vi "PicoScope5000aGetTimebase2.vi"(4 "Number of Samples":u32, 6 "Memory Segment":u32, 7 "Acquisition Settings":T2={"preTriggerSamples"=0, "postTriggerSamples"=1000, "timebase"=2, "Down-Sample Mode"=0, "Down Sample Ratio"=1} {"Down Sample Ratio" min=1 step=1; "Down-Sample Mode" items=["None"=0, "Aggregate"=1, "Decimate"=2, "Average"=4]}, 10 "handle in":i16, 11 "error in (no error)":errorcluster) -> (2 "handle out":i16, 3 "error out":errorcluster, 5 "Properties Panel":T1 {"Max Total Capture Time Available (sec)" format="%.3p"; "Sample Frequency" format="%.3p"; "Sample Rate" format="%.3p"; "Max Samples Available" format="%.3p"; "Total Capture Time (sec)" format="%.3p"})   [LabVIEW 2020]
uses:
  ps5000a.dll
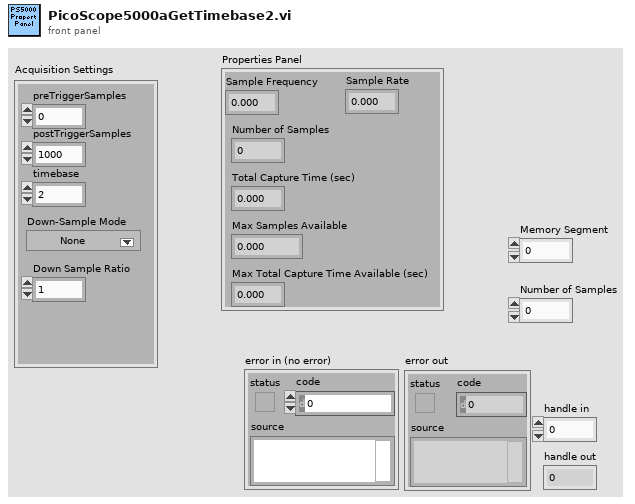
[diagram p1: front panel]
types:
  T1 = cluster{"Sample Frequency":sgl, "Sample Rate":sgl, "Max Samples Available":i32, "Number of Samples":u32, "Total Capture Time (sec) ":sgl, "Max Total Capture Time Available (sec)":sgl}
  T2 = cluster{"preTriggerSamples":i32, "postTriggerSamples":i32, "timebase":u32, "Down-Sample Mode":u32, "Down Sample Ratio":u32}
  T3 = cluster{sgl, sgl, "maxSamples":i32, "Number of Samples":u32, sgl, sgl}
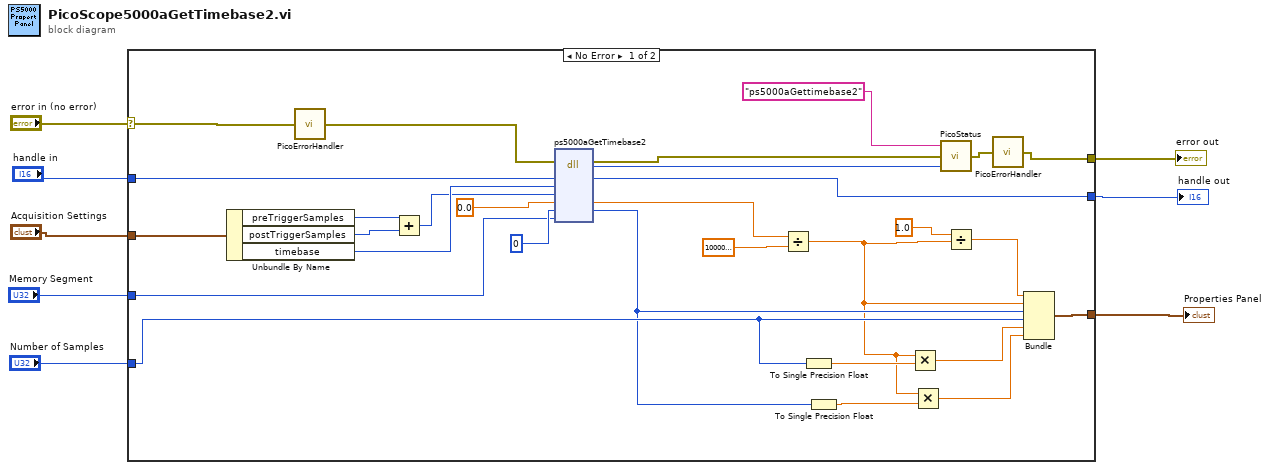
[diagram p0: block diagram]
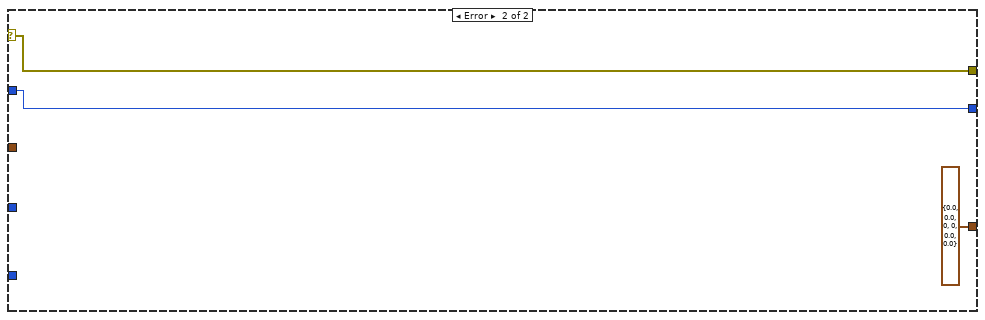
[diagram p2: hidden frame]
diagram:
  n1 = case shown="No Error" "error in (no error)" {
    selector: "error in (no error)" -> [w26 w40]
    tunnel: [w9 w40] -> w8
    tunnel: [w25 w39] -> w7
    tunnel: "Memory Segment" -> [w24 _]
    tunnel: "Number of Samples" -> [w18 _]
    tunnel: "handle in" -> [w23 w39]
    tunnel: "Acquisition Settings" -> [w22 _]
    tunnel: [w14 T3 {0.0, 0.0, "maxSamples"=0, "Number of Samples"=0, 0.0, 0.0}] -> w1
    frame No Error {
      n2 = Unbundle By Name(w22) -> ("preTriggerSamples"=w31:i32, "postTriggerSamples"=w32:i32, "timebase"=w33:u32)
      n3 = call "PicoErrorHandler.vi"("error in"=w26) -> ("error out"=w35:errorcluster)
      n4 = Add(x=w31, y=w32) -> (x+y=w20:i32)
      n5 = dll-call lib="ps5000a.dll" fn="ps5000aGetTimebase2"(error in=w35, "handle"=w23, "timebase"=w33, "noSamples"=w20, "timeIntervalNanoseconds"=sgl 0.0, "maxSamples"=0, "segmentIndex"=w24) -> (error out=w34:errorcluster, "PICO_STATUS"=w27:u32, "handle"=w25:i16, "timeIntervalNanoseconds"=w36:sgl, "maxSamples"=w16:i32)  [unwired: 5 in, 1 out]
      n6 = Divide(x=w36, y=sgl 1000000000.0) -> (x/y=w13:sgl)
      n7 = To Single Precision Float(number=w18) -> (single precision float=w21:sgl)
      n8 = To Single Precision Float(number=w16) -> (single precision float=w17:sgl)
      n9 = Multiply(x=w13, y=w21) -> (x*y=w19:sgl)
      n10 = Multiply(x=w13, y=w17) -> (x*y=w15:sgl)
      n11 = call "PicoStatus.vi"("PICO STATUS"=w27, "error in"=w34, "source"="ps5000aGettimebase2") -> ("error out"=w10:errorcluster)
      n12 = Divide(x=sgl 1.0, y=w13) -> (x/y=w11:sgl)
      n13 = call "PicoErrorHandler.vi"("error in"=w10) -> ("error out"=w9:errorcluster)
      n14 = Bundle(w11, w13, "maxSamples"=w16, "Number of Samples"=w18, w19, w15) -> (w14:T3)  [unwired: 1 in]
    }
    frame Error {
    }
  }
  "error out" <- w8
  "handle out" <- w7
  "Properties Panel" <- w1
